vi "UtilsStr_DeleteInString.vi"(2 "StringsToDelete":string[](array[string]), 3 "InputString":string) -> (1 "OutputString":string)   [LabVIEW 2013]
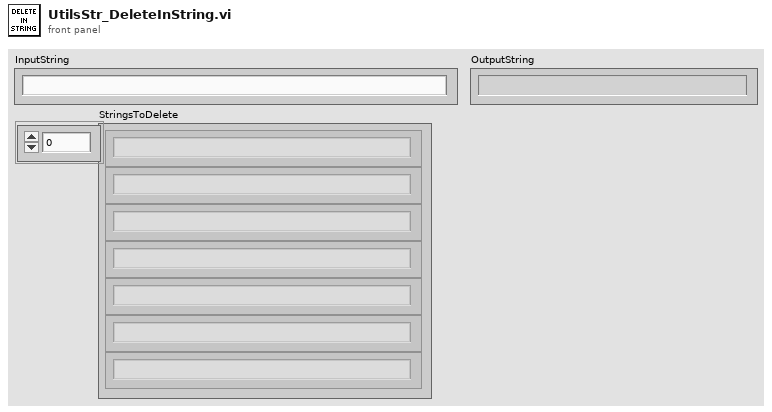
[diagram p1: front panel]
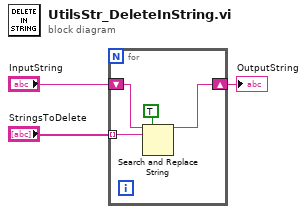
[diagram p0: block diagram]
diagram:
  n1 = for {
    shift-right: [w4] -> w1
    shift-left: "InputString" -> [w6]
    tunnel: "StringsToDelete" -> [w5] mode=indexing
    n2 = Search and Replace String(replace all?=TRUE ("tout remplacer ? (F)"), input string=w6, search string=w5) -> (result string=w4:string)  [unwired: 5 in, 3 out]
  }
  "OutputString" <- w1
